vi "pickKeeperRobots.vi"(8 "error in (no error)":errorcluster, 11 "Game in":refnum<class "Game.lvclass">) -> (0 "error out":errorcluster, 3 "Game out":refnum<class "Game.lvclass">)   [LabVIEW 2018, in "Game.lvclass"]
uses:
  Game.lvclass
  Game.lvclass/Game.ctl
  Team_class/Team.lvclass/Team.ctl
  Playbook_class/Playbook.lvclass/Playbook.ctl
  TestPlay_class/TestPlay.lvclass/TestPlay.ctl
  Robot_class/roles.ctl
  Role_class/Role.lvclass/Role.ctl
  Robot_class/Robot.lvclass/Robot.ctl
  HaltPlay_class/HaltPlay.lvclass/HaltPlay.ctl
  Robot_class/Write role.vi
  TestPlay_class/Read Roles.vi
  Role_class/Write RobotRef.vi
  TestPlay_class/Write Roles.vi
  Playbook_class/Write keeper_plays.vi
  Playbook_class/Read keeper_plays.vi
  TestPlay_class/Read NumberOfRobots.vi
  HaltPlay_class/Read Roles.vi
  HaltPlay_class/Write Roles.vi
  HaltPlay_class/Read NumberOfRobots.vi
  Read AllyRef.vi
  Read Referee.vi
  Read Playbook.vi
  Read KeeperTeam.vi
  Team_class/Read KeeperPlay.vi
  Team_class/Read RobotRef.vi
  Team_class/Write RobotRef.vi
  Write KeeperTeam.vi
  Write Playbook.vi
  Ally_class/Ally.lvclass
  C:/Users/nicolas.oliveira/roboime/SSL_AI/Team_class/Team.lvclass
  TestRole_class/TestRole.lvclass
  C:/Users/nicolas.oliveira/roboime/SSL_AI/Role_class/Role.lvclass
  HaltRole_class/HaltRole.lvclass
  Referee_class/Referee.lvclass
  Playbook_class/Playbook.lvclass
  Robot_class/Robot.lvclass
  Play_class/Play.lvclass
  TestPlay_class/TestPlay.lvclass
  HaltPlay_class/HaltPlay.lvclass
  Role_class/Role.lvclass
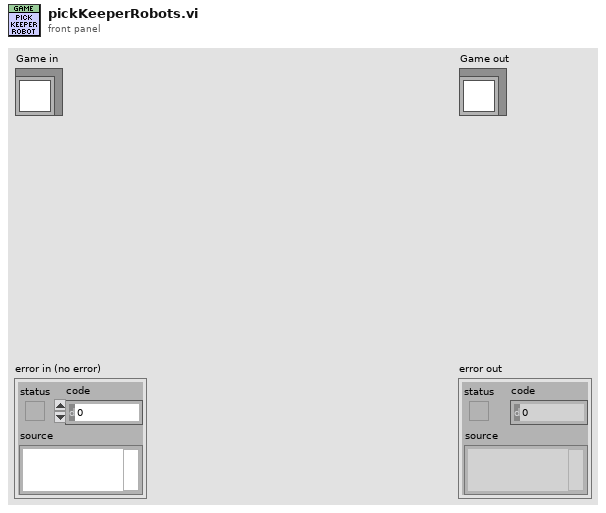
[diagram p1: front panel]
types:
  T1 = typedef "roles.ctl" = enum16{"Halt", "Role", "TestRole"}
  T2 = typedef "KeeperPlay.ctl" = enum16{"NormalGame", "Halt", "Timeout", "PenaltyEnemy", "TestPlay"}
  T3 = cluster{"Play":refnum<class "Play.lvclass">, "TestPlay":refnum<class "TestPlay.lvclass">, "HaltPlay":refnum<class "HaltPlay.lvclass">}
  T4 = cluster{"TestRole":refnum<class "TestRole.lvclass">, "Role":refnum<class "Role.lvclass">}
  T5 = cluster{"HaltRole":refnum<class "HaltRole.lvclass">}
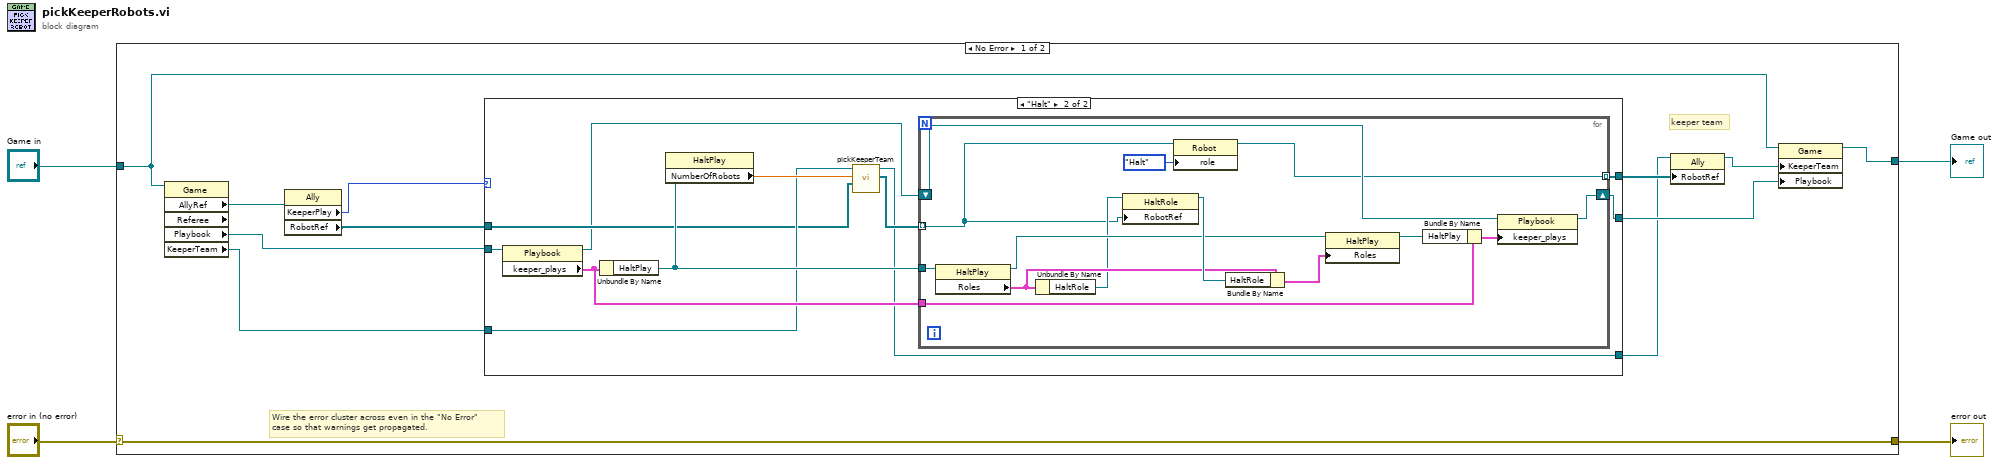
[diagram p0: block diagram]
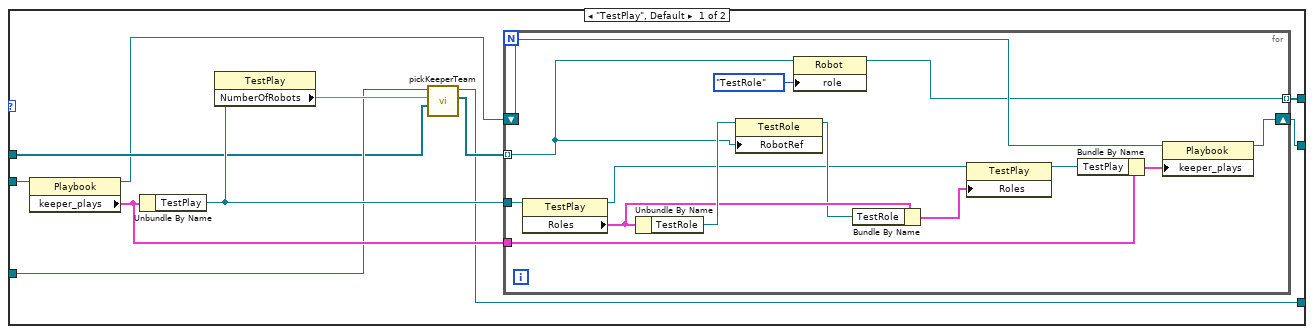
[diagram p2: hidden frame]
diagram:
  n1 = case shown="No Error" "error in (no error)" {
    selector: "error in (no error)" -> [w9 w68]
    tunnel: [w9 w68] -> w3
    tunnel: [w10 w67] -> w1
    tunnel: "Game in" -> [w12 w67]
    frame No Error {
      # "keeper team"
      # "Wire the error cluster across even in the \"No Error\"\ncase so that warnings get propagated."
      n2 = property class="Game" props=["AllyRef", "Referee", "Playbook", "KeeperTeam"](reference=w12) -> ("AllyRef"=w16:refnum<class "Ally.lvclass">, "Playbook"=w14:refnum<class "Playbook.lvclass">, "KeeperTeam"=w7:refnum<class "Ally.lvclass">)  [unwired: 1 in, 3 out]
      n3 = property class="Ally"(reference=w16) -> ("KeeperPlay"=w15:T2, "RobotRef"=w13:refnum<class "Robot.lvclass">[])  [unwired: 1 in, 2 out]
      n4 = case shown="\"Halt\"" w15 {
        tunnel: w14 -> [w27 w52]
        tunnel: w13 -> [w20 w45]
        tunnel: [w25 w50] -> w11
        tunnel: [w24 w49] -> w6
        tunnel: w7 -> [w21 w46]
        tunnel: [w17 w42] -> w5
        frame "TestPlay", Default {
          n5 = property class="Playbook"(reference=w27) -> (reference out=w19:refnum<class "Playbook.lvclass">, "keeper_plays"=w26:T3)  [unwired: 1 in, 1 out]
          n6 = Unbundle By Name(w26) -> ("TestPlay"=w23:refnum<class "TestPlay.lvclass">)
          n7 = property class="TestPlay"(reference=w23) -> ("NumberOfRobots"=w22:dbl)  [unwired: 1 in, 2 out]
          n8 = call-dynamic "pickKeeperTeam.vi"("RobotRef"=w20, "number_of_robots"=w22, "Ally in"=w21) -> ("RobotRef out"=w18:refnum<class "Robot.lvclass">[], "Ally out"=w17:refnum<class "Ally.lvclass">)  [unwired: 6 in, 1 out]
          n9 = for {
            tunnel: w26 -> [w36]
            tunnel: [w29] -> w24 mode=indexing
            tunnel: w23 -> [w30]
            tunnel: w18 -> [w28] mode=indexing
            shift-right: [w32] -> w25
            shift-left: w19 -> [w33]
            n10 = property class="TestPlay"(reference=w30) -> (reference out=w37:refnum<class "TestPlay.lvclass">, "Roles"=w40:T4)  [unwired: 1 in, 1 out]
            n11 = Unbundle By Name(w40) -> ("TestRole"=w41:refnum<class "TestRole.lvclass">)
            n12 = property class="TestRole"(reference=w41, "RobotRef"=w28) -> (reference out=w39:refnum<class "TestRole.lvclass">)  [unwired: 1 in, 1 out]
            n13 = property class="Robot"(reference=w28, "role"=roles."TestRole") -> (reference out=w29:refnum<class "Robot.lvclass">)  [unwired: 1 in, 1 out]
            n14 = Bundle By Name(cluster=w40, "TestRole"=w39) -> (w38:T4)
            n15 = property class="TestPlay"(reference=w37, "Roles"=w38) -> (reference out=w35:refnum<class "TestPlay.lvclass">)  [unwired: 1 in, 1 out]
            n16 = Bundle By Name(cluster=w36, "TestPlay"=w35) -> (w34:T3)
            n17 = property class="Playbook"(reference=w33, "keeper_plays"=w34) -> (reference out=w32:refnum<class "Playbook.lvclass">)  [unwired: 1 in, 1 out]
          }
        }
        frame "Halt" {
          n18 = property class="Playbook"(reference=w52) -> (reference out=w44:refnum<class "Playbook.lvclass">, "keeper_plays"=w51:T3)  [unwired: 1 in, 1 out]
          n19 = Unbundle By Name(w51) -> ("HaltPlay"=w48:refnum<class "HaltPlay.lvclass">)
          n20 = property class="HaltPlay"(reference=w48) -> ("NumberOfRobots"=w47:dbl)  [unwired: 1 in, 2 out]
          n21 = call-dynamic "pickKeeperTeam.vi"("RobotRef"=w45, "number_of_robots"=w47, "Ally in"=w46) -> ("RobotRef out"=w43:refnum<class "Robot.lvclass">[], "Ally out"=w42:refnum<class "Ally.lvclass">)  [unwired: 6 in, 1 out]
          n22 = for {
            tunnel: w51 -> [w63]
            tunnel: [w57] -> w49 mode=indexing
            tunnel: w48 -> [w58]
            tunnel: w43 -> [w53] mode=indexing
            shift-right: [w59] -> w50
            shift-left: w44 -> [w60]
            n23 = property class="HaltPlay"(reference=w58) -> (reference out=w64:refnum<class "HaltPlay.lvclass">, "Roles"=w56:T5)  [unwired: 1 in, 1 out]
            n24 = Unbundle By Name(w56) -> ("HaltRole"=w55:refnum<class "HaltRole.lvclass">)
            n25 = property class="HaltRole"(reference=w55, "RobotRef"=w53) -> (reference out=w66:refnum<class "HaltRole.lvclass">)  [unwired: 1 in, 1 out]
            n26 = property class="Robot"(reference=w53, "role"=roles."Halt") -> (reference out=w57:refnum<class "Robot.lvclass">)  [unwired: 1 in, 1 out]
            n27 = Bundle By Name(cluster=w56, "HaltRole"=w66) -> (w65:T5)
            n28 = property class="HaltPlay"(reference=w64, "Roles"=w65) -> (reference out=w62:refnum<class "HaltPlay.lvclass">)  [unwired: 1 in, 1 out]
            n29 = Bundle By Name(cluster=w63, "HaltPlay"=w62) -> (w61:T3)
            n30 = property class="Playbook"(reference=w60, "keeper_plays"=w61) -> (reference out=w59:refnum<class "Playbook.lvclass">)  [unwired: 1 in, 1 out]
          }
        }
      }
      n31 = property class="Ally"(reference=w5, "RobotRef"=w6) -> (reference out=w8:refnum<class "Ally.lvclass">)  [unwired: 1 in, 1 out]
      n32 = property class="Game"(reference=w12, "KeeperTeam"=w8, "Playbook"=w11) -> (reference out=w10:refnum<class "Game.lvclass">)  [unwired: 1 in, 1 out]
    }
    frame Error {
    }
  }
  "error out" <- w3
  "Game out" <- w1
